vi "Identify.vi"(8 "error in (no error)":errorcluster, 11 "ModSweep in":refnum<class "ModSweep.lvclass">) -> (0 "error out":errorcluster, 2 "Plugin is Valid":bool, 3 "ModSweep out":refnum<class "ModSweep.lvclass">)   [LabVIEW 2018, in "ModSweep.lvlib" / "ModSweep.lvclass"]
uses:
  ModSweep.lvclass
  C:/Sequence Automation/Plugins/Measurement Interface.lvlibp/Measurement Interface.lvclass
  Plugins/Measurement Interface.lvlibp/Private Methods/Measurement Definition Entry/Read Measurement Definition Entry.vi
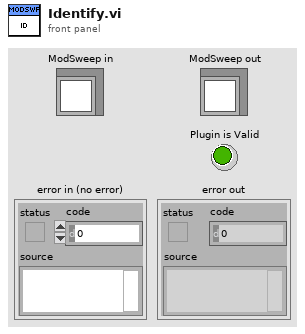
[diagram p1: front panel]
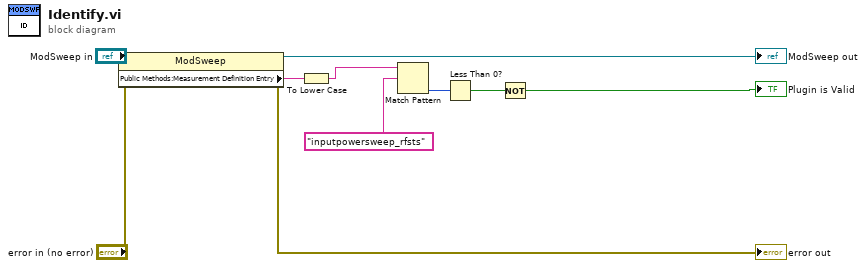
[diagram p0: block diagram]
diagram:
  n1 = property class="ModSweep"(reference="ModSweep in", error in="error in (no error)") -> (reference out=→"ModSweep out":refnum<class "ModSweep.lvclass">, error out=→"error out":errorcluster, "Public Methods:Measurement Definition Entry"=w6:string)
  n2 = To Lower Case(string=w6) -> (all lower case string=w4:string)
  n3 = Match Pattern(string=w4, regular expression="inputpowersweep_rfsts" ("y")) -> (offset past match=w2:i32)  [unwired: 1 in, 3 out]
  n4 = Less Than 0?(x=w2) -> (x < 0?=w5:bool)
  n5 = Not(x=w5) -> (.not. x?=→"Plugin is Valid":bool)
